vi "Get Timing Section.vi"(8 "error in":errorcluster, 11 "custom device in":T1 format="%.0x") -> (0 "error out":errorcluster, 2 "timing section out":T1 format="%.0x", 3 "custom device out":T1 format="%.0x", 4 "found":bool)   [LabVIEW 2020, in "Ballard MIL-STD-1553 Scripting.lvlib"]
uses:
  Ballard MIL-STD-1553 Scripting.lvlib
  <vilib>/NI VeriStand/Custom Device Tools/Custom Device Utility Library/Custom Device Utility Library.lvlib
  <vilib>/NI VeriStand/Custom Device Tools/Custom Device Utility Library/NI VeriStand - Search for Item by GUID.vi
  Constants.vi
  <vilib>/NI VeriStand/Custom Device API/Custom Device Item Ref.ctl
  <vilib>/NI VeriStand/Custom Device API/Custom Device API.lvlib
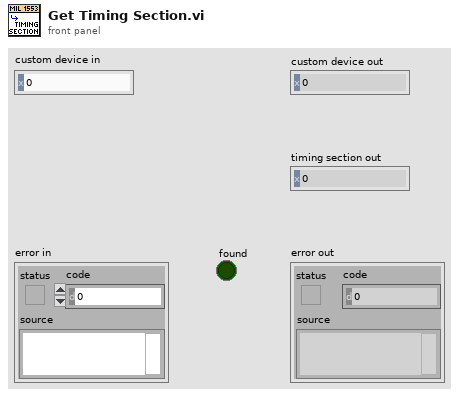
[diagram p1: front panel]
types:
  T1 = typedef "Custom Device API.lvlib/Custom Device Item Ref.ctl" = u64
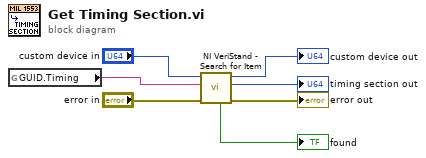
[diagram p0: block diagram]
diagram:
  n1 = global read "Constants.vi" "GUID.Timing"() -> (w2:string)
  n2 = call-poly <vilib>:"NI VeriStand - Search for Item.vi"("error in"="error in", "Item GUID"=w2, "Section Ref in"="custom device in") -> ("error out"=→"error out":errorcluster, "Item Ref"=→"timing section out":T1, "Section Ref out"=→"custom device out":T1, "Found"=→"found":bool)  [unwired: 5 in]
